vi "Configure Measuring Parameters.vi"(0 "VISA resource name":refnum<visa-resource-name>, 1 "range (1 ohm:1)":u16(ring)=1 items=["0.1 ohms", "1 ohm", "10 ohms", "100 ohms", "1k ohms", "10k ohms", "100k ohms", "1M ohms"], 5 "Auto Range (T)":bool=TRUE, 9 "Enable contact check (F)":bool, 11 "error in (no error)":errorcluster, 12 "aperture (short:0)":u16(ring) items=["short (0.025 sec)", "medium (0.065 sec)", "long (0.500 sec)"]) -> (4 "VISA resource name out":refnum<visa-resource-name>, 15 "error out":errorcluster)   [LabVIEW 2016, in "Agilent 4263X.lvlib"]
doc: "This VI configures the measurment parameters of the instrument."
uses:
  <instrlib>/Agilent 4263X/Agilent 4263X.lvlib
panel:
  # "on\noff"
  # "on\noff"
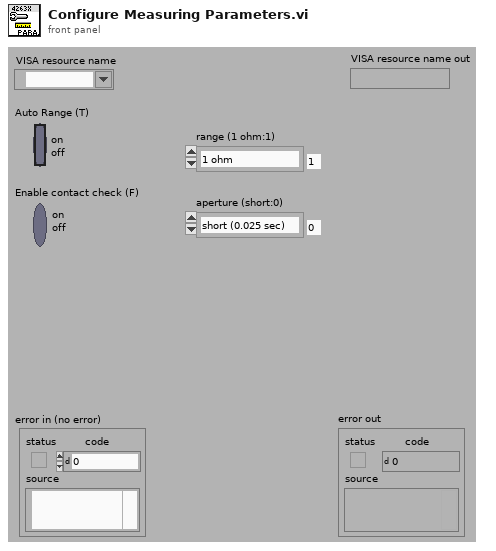
[diagram p1: front panel]
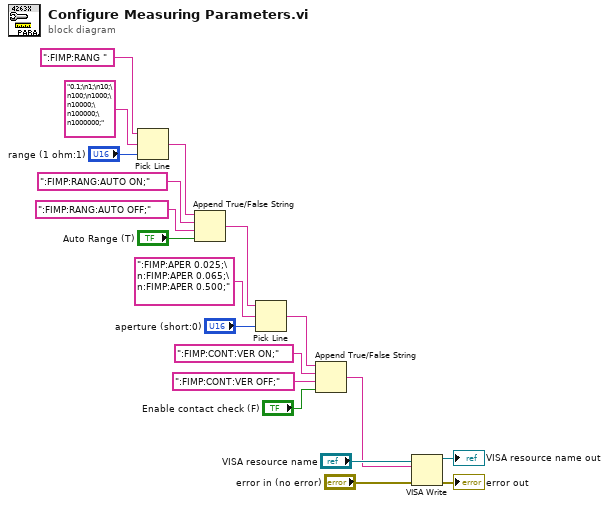
[diagram p0: block diagram]
diagram:
  n1 = Pick Line(string ("")=":FIMP:RANG ", multi-line string="0.1;\n1;\n10;\n100;\n1000;\n10000;\n100000;\n1000000;", line index="range (1 ohm:1)") -> (output string=w2:string)
  n2 = Append True/False String(1:"Auto Range (T)", 2:":FIMP:RANG:AUTO OFF;", 3:":FIMP:RANG:AUTO ON;", 4:w2) -> (0:w1:string)
  n3 = Pick Line(string ("")=w1, multi-line string=":FIMP:APER 0.025;\n:FIMP:APER 0.065;\n:FIMP:APER 0.500;", line index="aperture (short:0)") -> (output string=w9:string)
  n4 = Append True/False String(1:"Enable contact check (F)", 2:":FIMP:CONT:VER OFF;", 3:":FIMP:CONT:VER ON;", 4:w9) -> (0:w5:string)
  n5 = VISA Write(VISA resource name="VISA resource name", write buffer=w5, error in (no error)="error in (no error)") -> (VISA resource name out=→"VISA resource name out":refnum<visa-resource-name>, error out=→"error out":errorcluster)  [unwired: 1 out]
